vi "Find Standard Deviation of the First N Entries of an Array.vi"(10 "N":u32, 11 "Array":sgl[](array[numeric])) -> (2 "standard deviation":dbl)   [LabVIEW 2013]
uses:
  <vilib>/Analysis/NI_AALBase.lvlib
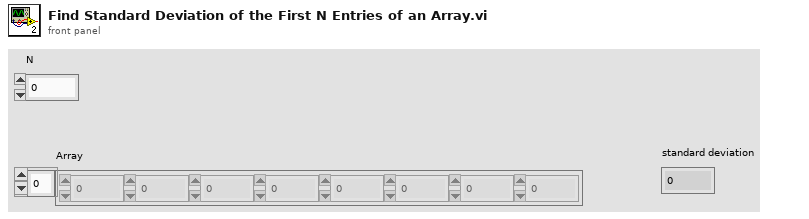
[diagram p1: front panel]
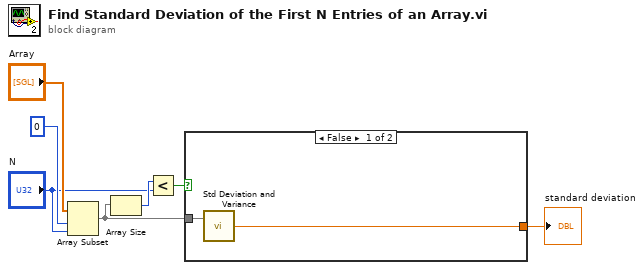
[diagram p0: block diagram]
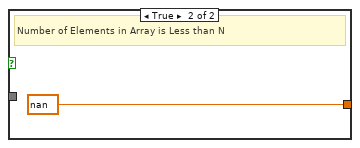
[diagram p2: hidden frame]
diagram:
  n1 = Array Subset(array="Array", index=0, length="N") -> (w2:sgl[])
  n2 = Array Size(array=w2) -> (size(s)=w5:i32)
  n3 = Less?(x=w5, y="N") -> (x < y?=w3:bool)
  n4 = case shown="False" w3 {
    tunnel: w2 -> [w9 _]
    tunnel: [w8 nan ("standard deviation")] -> w1
    frame False {
      n5 = call <vilib>:"Std Deviation and Variance.vi"("X"=w9) -> ("standard deviation"=w8:dbl)  [unwired: 1 in, 2 out]
    }
    frame True {
      # "Number of Elements in Array is Less than N"
    }
  }
  "standard deviation" <- w1
